vi "CSM Execute - Interface Browser.vi"(6 "Mouse Position":T1, 8 "User VI Ref":refnum<vi>, 9 "Menu Item Tag Suffix":string, 10 "Remaining Items":refnum<vi>[](array[refnum]), 11 "Affected Items":T2) -> (0 "Fail transaction?":bool)   [LabVIEW 2017]
doc: "This VI is part of a plug-in for modifying the LabVIEW shortcut menus. This is the execute VI which is called when the shortcut menu is chosen by the user. It performs the action of the selected menu item."
uses:
  CSM Execute - Shortcut Menu Plug-In.ctl
  <vilib>/Utility/miscctls.llb/LVPositionTypeDef.ctl
panel:
  # "All controls on this panel except \"Affected Items\" have been locked to prevent accidental edits. Changing the control names or types, other than the elements of the \"Affected Items\" cluster will make the VI unusable as a menu plugin.\n\nSee Context Help for each control for details about its use."
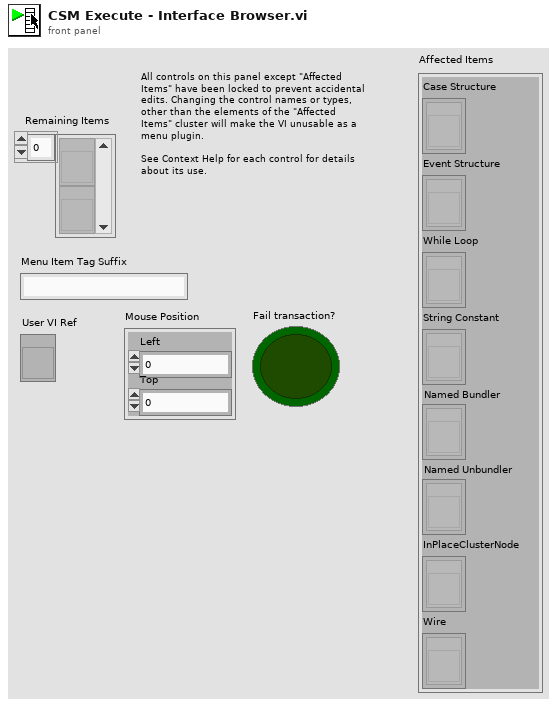
[diagram p1: front panel]
types:
  T1 = typedef "LVPositionTypeDef.ctl" = cluster{"Left":i32, "Top":i32}
  T2 = typedef "CSM Execute - Shortcut Menu Plug-In.ctl" = cluster{"Case Structure":refnum<vi>[], "Event Structure":refnum<vi>[], "While Loop":refnum<vi>[], "String Constant":refnum<vi>[], "Named Bundler":refnum<vi>[], "Named Unbundler":refnum<vi>[], "InPlaceClusterNode":refnum<vi>[], "Wire":refnum<vi>[]}
  T3 = typedef "LVRectTypeDef.ctl" = cluster{"Left":i16, "Top":i16, "Right":i16, "Bottom":i16}
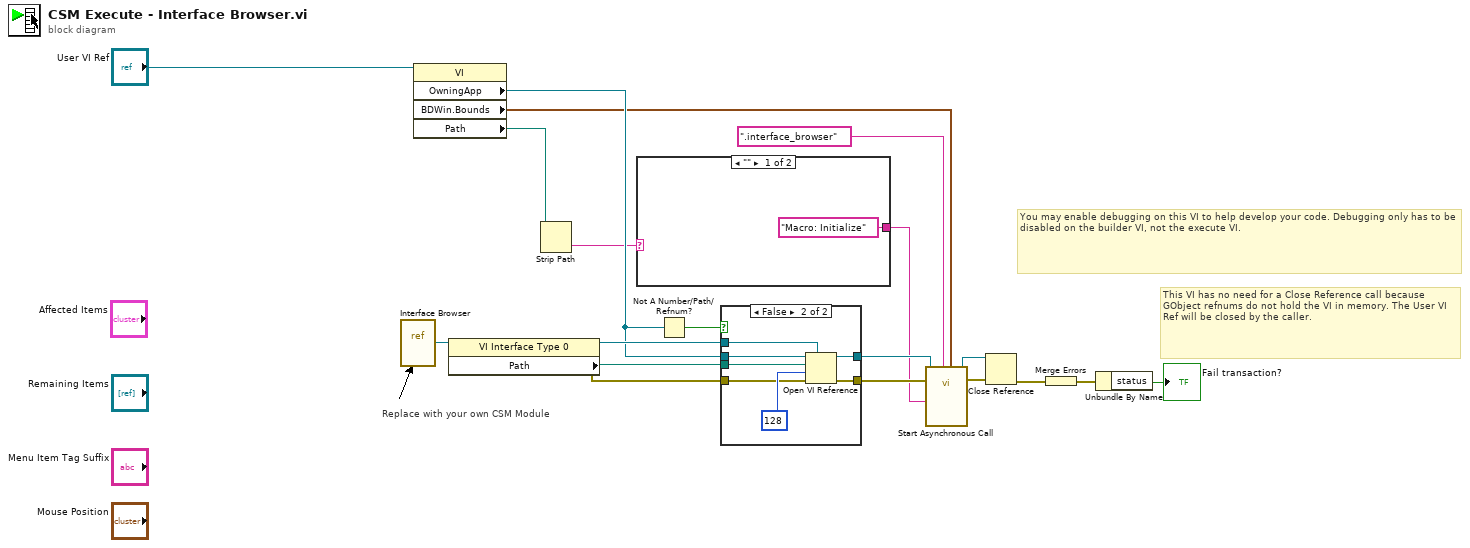
[diagram p0: block diagram]
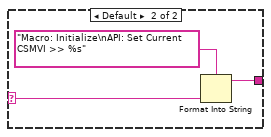
[diagram p2: hidden frame]
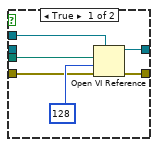
[diagram p3: hidden frame]
diagram:
  # "Replace with your own CSM Module"
  # "You may enable debugging on this VI to help develop your code. Debugging only has to be disabled on the builder VI, not the execute VI."
  # "This VI has no need for a Close Reference call because GObject refnums do not hold the VI in memory. The User VI Ref will be closed by the caller."
  n1 = vi-ref "Interface Browser.vi"() -> (w11:refnum<vi>)
  n2 = property class="VI"(reference="User VI Ref") -> ("OwningApp"=w5:refnum<vi>, "BDWin.Bounds"=w4:T3, "Path"=w3:path)  [unwired: 1 in, 2 out]
  n3 = property class="VI Interface Type 0"(reference=w11) -> (reference out=w15:refnum<vi>, error out=w13:errorcluster, "Path"=w12:path)  [unwired: 1 in]
  n4 = Strip Path(path=w3) -> (name=w2:string)  [unwired: 1 out]
  n5 = case shown="\"\"" w2 {
    selector: w2 -> [_ w22]
    tunnel: ["Macro: Initialize" w21] -> w1
    frame "" {
    }
    frame Default {
      n6 = Format Into String(format string="Macro: Initialize\nAPI: Set Current CSMVI >> %s" ("Init State(\"Macro: Initialize\")"), w22) -> (resulting string=w21:string)  [unwired: 2 in, 1 out]
    }
  }
  n7 = Not A Number/Path/Refnum?(number/path/refnum=w5) -> (NaN/Path/Refnum?=w6:bool)
  n8 = case shown="False" w6 {
    tunnel: w15 -> [w28 w35]
    tunnel: [w27 w34] -> w14
    tunnel: w13 -> [w26 w33]
    tunnel: w12 -> [w25 w32]
    tunnel: [w24 w31] -> w10
    tunnel: w5 -> [_ w30]
    frame True {
      n9 = Open VI Reference(type specifier VI Refnum (for type only)=w28, vi path=w25, options=128, error in (no error)=w26) -> (vi reference=w27:refnum<vi>, error out=w24:errorcluster)  [unwired: 2 in]
    }
    frame False {
      n10 = Open VI Reference(type specifier VI Refnum (for type only)=w35, application reference (local)=w30, vi path=w32, options=128, error in (no error)=w33) -> (vi reference=w34:refnum<vi>, error out=w31:errorcluster)  [unwired: 1 in]
    }
  }
  n11 = call-by-ref "Start Asynchronous Call"(reference=w14, error in=w10, "Caller Window Bounds"=w4, "Name(\"\" to use uuid)"=".interface_browser" ("Name(\"\" to use uuid)"), "Init State(\"Macro: Initialize\")"=w1) -> (reference out=w17:refnum<vi>, error out=w16:errorcluster)  [unwired: 9 in]
  n12 = Close Reference(reference=w17, error in (no error)=w16) -> (error out=w9:errorcluster)
  n13 = Merge Errors(w9) -> (w18:errorcluster)
  n14 = Unbundle By Name(w18) -> ("status"=→"Fail transaction?":bool)
